vi "1 Channel 1 Sample - Auto Indexing.vi"() -> ()   [LabVIEW 2026, in "synnax_clib.lvlib"]
uses:
  typedefs/connection_config.ctl
  classes/Client/Private/synnax channel retrieve keys Single.vi
  classes/Writer/Private/synnax writer open Single.vi
  classes/Writer/Private/Writes/DBL/Write 1Ch 1Samp (DBL).vi
  synnax_clib.lvlib
  classes/Synnax Writer.lvclass
  classes/Client/Synnax Client.lvclass
panel:
  out "cos(x)":dbl
  in  "Stop":bool
  out "error out":errorcluster
  in  "Channel":string="my_f64_chan"
  in  "Connection Config":T1={"host"="localhost", "port"=9090, "username"="synnax", "password"="seldon"}
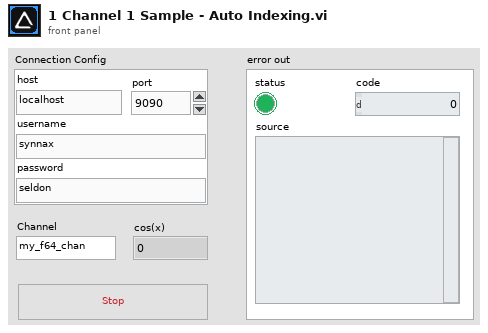
[diagram p1: front panel]
types:
  T1 = typedef "synnax_clib.lvlib/connection_config.ctl" = cluster{"host":string, "port":u16, "username":string, "password":string}
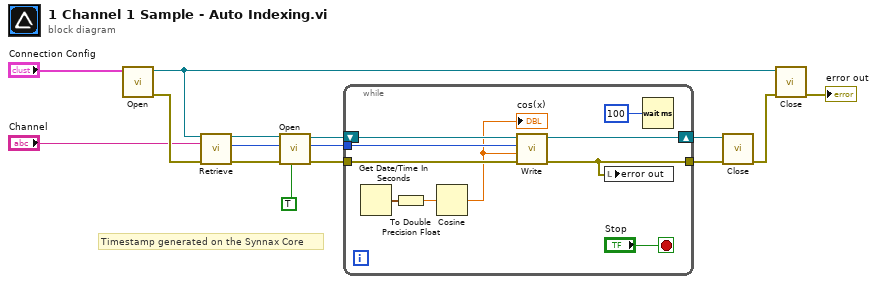
[diagram p0: block diagram]
diagram:
  # "Timestamp generated on the Synnax Core"
  n1 = call "Open.vi"("Connection Config"="Connection Config") -> ("error out"=w10:errorcluster, "Synnax Client out"=w12:refnum<class "Synnax Client.lvclass">)  [unwired: 9 in]
  n2 = call-poly "Retrieve.vi"("Synnax Client in"=w12, "channel name"="Channel", "error in"=w10) -> ("Synnax Client out"=w6:refnum<class "Synnax Client.lvclass">, "channel key"=w2:u32, "error out"=w14:errorcluster)  [unwired: 9 in, 1 out]
  n3 = call-poly "Open.vi"("auto_index (F)"=TRUE, "error in"=w14, "channel in"=w2, "Synnax Client in"=w6) -> ("error out"=w7:errorcluster, "channel out"=w3:u32, "writer out"=w9:refnum<class "Synnax Writer.lvclass">)  [unwired: 5 in]
  n4 = while {
    tunnel: w3 -> [w22]
    shift-right: [w24] -> w8
    shift-left: w9 -> [w25]
    tunnel: w7 -> [w23]
    tunnel: [w18] -> w15
    stop <- "Stop" stop-if-true
    n5 = Get Date/Time In Seconds() -> (seconds since 1Jan1904=w17:timestamp)
    n6 = To Double Precision Float(number=w17) -> (double precision float=w16:dbl)
    n7 = Cosine(x=w16) -> (cos(x)=w20:dbl)
    "cos(x)" <- w20
    n8 = call-poly "Write.vi"("error in"=w23, "data"=w20, "channel"=w22, "Writer"=w25) -> ("error out"=w18:errorcluster, "Writer Out"=w24:refnum<class "Synnax Writer.lvclass">)  [unwired: 6 in]
    n9 = local write "error out"(w18) -> ()
    n10 = Wait (ms)(milliseconds to wait=u32 100) -> ()  [unwired: 1 out]
  }
  n11 = call "Close.vi"("error in"=w15, "writer"=w8) -> ("error out"=w11:errorcluster)  [unwired: 9 in]
  n12 = call "Close.vi"("error in"=w11, "Synnax Client in"=w12) -> ("error out"=→"error out":errorcluster)  [unwired: 9 in]
